vi "sortPhase (SubVI).vi"(11 "sortMag":T2(array[cluster])) -> (3 "sortPhase":T1(array[cluster]))   [LabVIEW 2011]
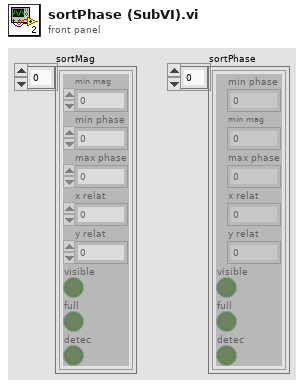
[diagram p1: front panel]
types:
  T1 = cluster{"min phase":dbl, "min mag":dbl, "max phase":dbl, "x relat":i32, "y relat":i32, "visible":bool, "full":bool, "detec":bool}[]
  T2 = cluster{"min mag":dbl, "min phase":dbl, "max phase":dbl, "x relat":i32, "y relat":i32, "visible":bool, "full":bool, "detec":bool}[]
  T3 = cluster{"min phase":dbl, "min mag":dbl, "max phase":dbl, "x relat":i32, "y relat":i32, "visible":bool, "full":bool, "detec":bool}
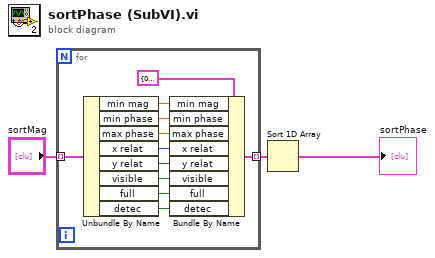
[diagram p0: block diagram]
diagram:
  n1 = for {
    tunnel: "sortMag" -> [w14] mode=indexing
    tunnel: [w4] -> w3 mode=indexing
    n2 = Unbundle By Name(w14) -> ("min mag"=w12:dbl, "min phase"=w11:dbl, "max phase"=w10:dbl, "x relat"=w9:i32, "y relat"=w8:i32, "visible"=w7:bool, "full"=w6:bool, "detec"=w5:bool)
    n3 = Bundle By Name(cluster=T3 {"min phase"=0.0, "min mag"=0.0, "max phase"=0.0, "x relat"=0, "y relat"=0, "visible"=FALSE, "full"=FALSE, "detec"=FALSE} ("output cluster"), "min mag"=w12, "min phase"=w11, "max phase"=w10, "x relat"=w9, "y relat"=w8, "visible"=w7, "full"=w6, "detec"=w5) -> (w4:T3)
  }
  n4 = Sort 1D Array(array=w3) -> (sorted array=→"sortPhase":T1)
